vi "Process Trigger.vi"(8 "error in (no error)":errorcluster, 9 "Trigger Values in":dbl[](array[numeric]), 11 "Trigger in":T1 {"Node Data Ref" format="%.0x"; "Node ID" format="%.0x"}) -> (0 "error out":errorcluster, 1 "Trigger Values out":dbl[](array[numeric]), 2 "Trigger":bool, 3 "Trigger out":T1 {"Node Data Ref" format="%.0x"; "Node ID" format="%.0x"})   [LabVIEW 2015, in "Waveform Data Logger Engine.lvlib"]
uses:
  Waveform Data Logger Engine.lvlib
  Types/Trigger Settings.ctl
  Classes/Triggers/Trigger/Trigger.lvclass
  <vilib>/NI Veristand/Custom Device API/Custom Device Item Ref.ctl
  Classes/Triggers/Trigger/Trigger.lvclass/Trigger.ctl
  Classes/Triggers/Digital Edge Trigger/Digital Edge Trigger.lvclass/Digital Edge Trigger.ctl
  Classes/Triggers/Analog Edge Trigger/Analog Edge Trigger.lvclass/Analog Edge Trigger.ctl
  Classes/Triggers/Value Change Trigger/Value Change Trigger.lvclass/Value Change Trigger.ctl
  Classes/Triggers/Boolean Evaluation Trigger/Boolean Evaluation Trigger.lvclass/Boolean Evaluation Trigger.ctl
  Classes/Triggers/Default Trigger/Default Trigger.lvclass/Default Trigger.ctl
  Classes/Triggers/Digital Edge Trigger/Evaluate Digital Edge Trigger.vi
  Classes/Triggers/Analog Edge Trigger/Evaluate Analog Edge Trigger.vi
  Classes/Triggers/Value Change Trigger/Evaluate Value Change Trigger.vi
  Classes/Triggers/Boolean Evaluation Trigger/Evaluate Boolean Evaluation Trigger.vi
  Classes/Triggers/Default Trigger/Evaluate Default Trigger.vi
  Classes/Triggers/In Range Trigger/Evaluate In Range Trigger.vi
  Classes/Triggers/Default Trigger/Default Trigger.lvclass
  Classes/Triggers/In Range Trigger/In Range Trigger.lvclass
  Classes/Triggers/Boolean Evaluation Trigger/Boolean Evaluation Trigger.lvclass
  Classes/Triggers/Value Change Trigger/Value Change Trigger.lvclass
  Classes/Triggers/Analog Edge Trigger/Analog Edge Trigger.lvclass
  Classes/Triggers/Digital Edge Trigger/Digital Edge Trigger.lvclass
  <vilib>/NI Veristand/Custom Device API/Custom Device API.lvlib
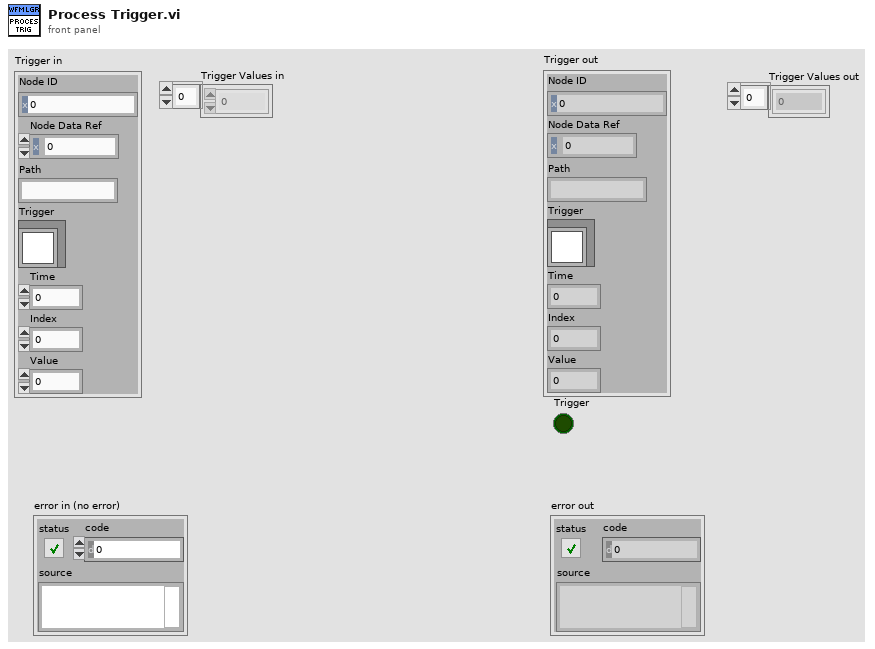
[diagram p1: front panel]
types:
  T1 = typedef "Waveform Data Logger Engine.lvlib/Trigger Settings.ctl" = cluster{"Node ID":T2, "Node Data Ref":i32, "Path":string, "Trigger":refnum<class "Trigger.lvclass">, "Time":dbl, "Index":i32, "Value":dbl}
  T2 = typedef "Custom Device API.lvlib/Custom Device Item Ref.ctl" = u64
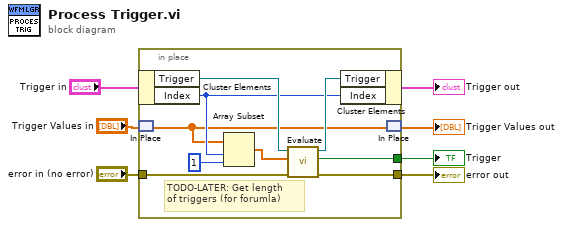
[diagram p0: block diagram]
diagram:
  n1 = in-place {
    in-place-border: "error in (no error)" -> [w16]
    in-place-border: [w15] -> w6
    in-place-border: [w14] -> w5
    # "TODO-LATER: Get length \nof triggers (for forumla)"
    n2 = in-place-cluster #1("Trigger in") -> ("Trigger"=w11:refnum<class "Trigger.lvclass">, "Index"=w9:i32)
    n3 = in-place-match #2("Trigger Values in") -> (w8:dbl[])
    n4 = Array Subset(array=w8, index=w9, length=1) -> (w12:dbl[])
    n5 = call "Evaluate.vi"("error in (no error)"=w16, "Trigger Data"=w12, "Trigger in"=w11) -> ("error out"=w14:errorcluster, "Trigger"=w15:bool, "Trigger out"=w10:refnum<class "Trigger.lvclass">)  [unwired: 6 in]
    n6 = in-place-cluster #1("Trigger"=w10, "Index"=w9) -> (→"Trigger out":T1)
    n7 = in-place-match #2(w8) -> (→"Trigger Values out":dbl[])
  }
  "Trigger" <- w6
  "error out" <- w5
